vi "SDF Small Gasifier RT - IO_backup.vi"(0 "CIE Tags":T1) -> ()   [LabVIEW 2013]
uses:
  <userlib>/CIE/_TypeDefs/CIE Tags.ctl
  <userlib>/CIE/_TypeDefs/DBL CIE Tag.ctl
  <userlib>/CIE/_TypeDefs/BOOL CIE Tag.ctl
  <userlib>/CIE/_TypeDefs/I32 CIE Tag.ctl
  <userlib>/CIE/_TypeDefs/Enum CIE Tag.ctl
  <userlib>/CIE/_TypeDefs/STR CIE Tag.ctl
  <vilib>/NI/Current Value Table/DataTypes/String_Read.vi
  <vilib>/NI/Current Value Table/DataTypes/Double_Read.vi
  <vilib>/NI/Current Value Table/DataTypes/Double_Write.vi
  <vilib>/NI/Current Value Table/DataTypes/Boolean_Write.vi
  <vilib>/NI/Current Value Table/Type to Enum.vi
  <vilib>/NI/Current Value Table/DataTypes/String_Type To Enum.vi
  <vilib>/NI/Current Value Table/DataTypes/Double_Type To Enum.vi
  <vilib>/NI/Current Value Table/DataTypes/Boolean_Type To Enum.vi
  <vilib>/NI/Current Value Table/FGVs/CVT Globals.vi
  <vilib>/NI/Current Value Table/FGVs/Tag Memory.vi
  <vilib>/NI/Current Value Table/Memory Block.vi
  <vilib>/NI/Current Value Table/DataTypes/String_Memory Block.vi
  <vilib>/NI/Current Value Table/DataTypes/Double_Memory Block.vi
  <vilib>/NI/Current Value Table/DataTypes/Boolean_Memory Block.vi
  <vilib>/NI/Current Value Table/Current Value Table.lvlib
panel:
  out "Missed Scan":bool
  out "Scan Error":errorcluster
  out "Value":string
  out "Numeric":dbl
  in  "Stop":bool
  out "Index":i32
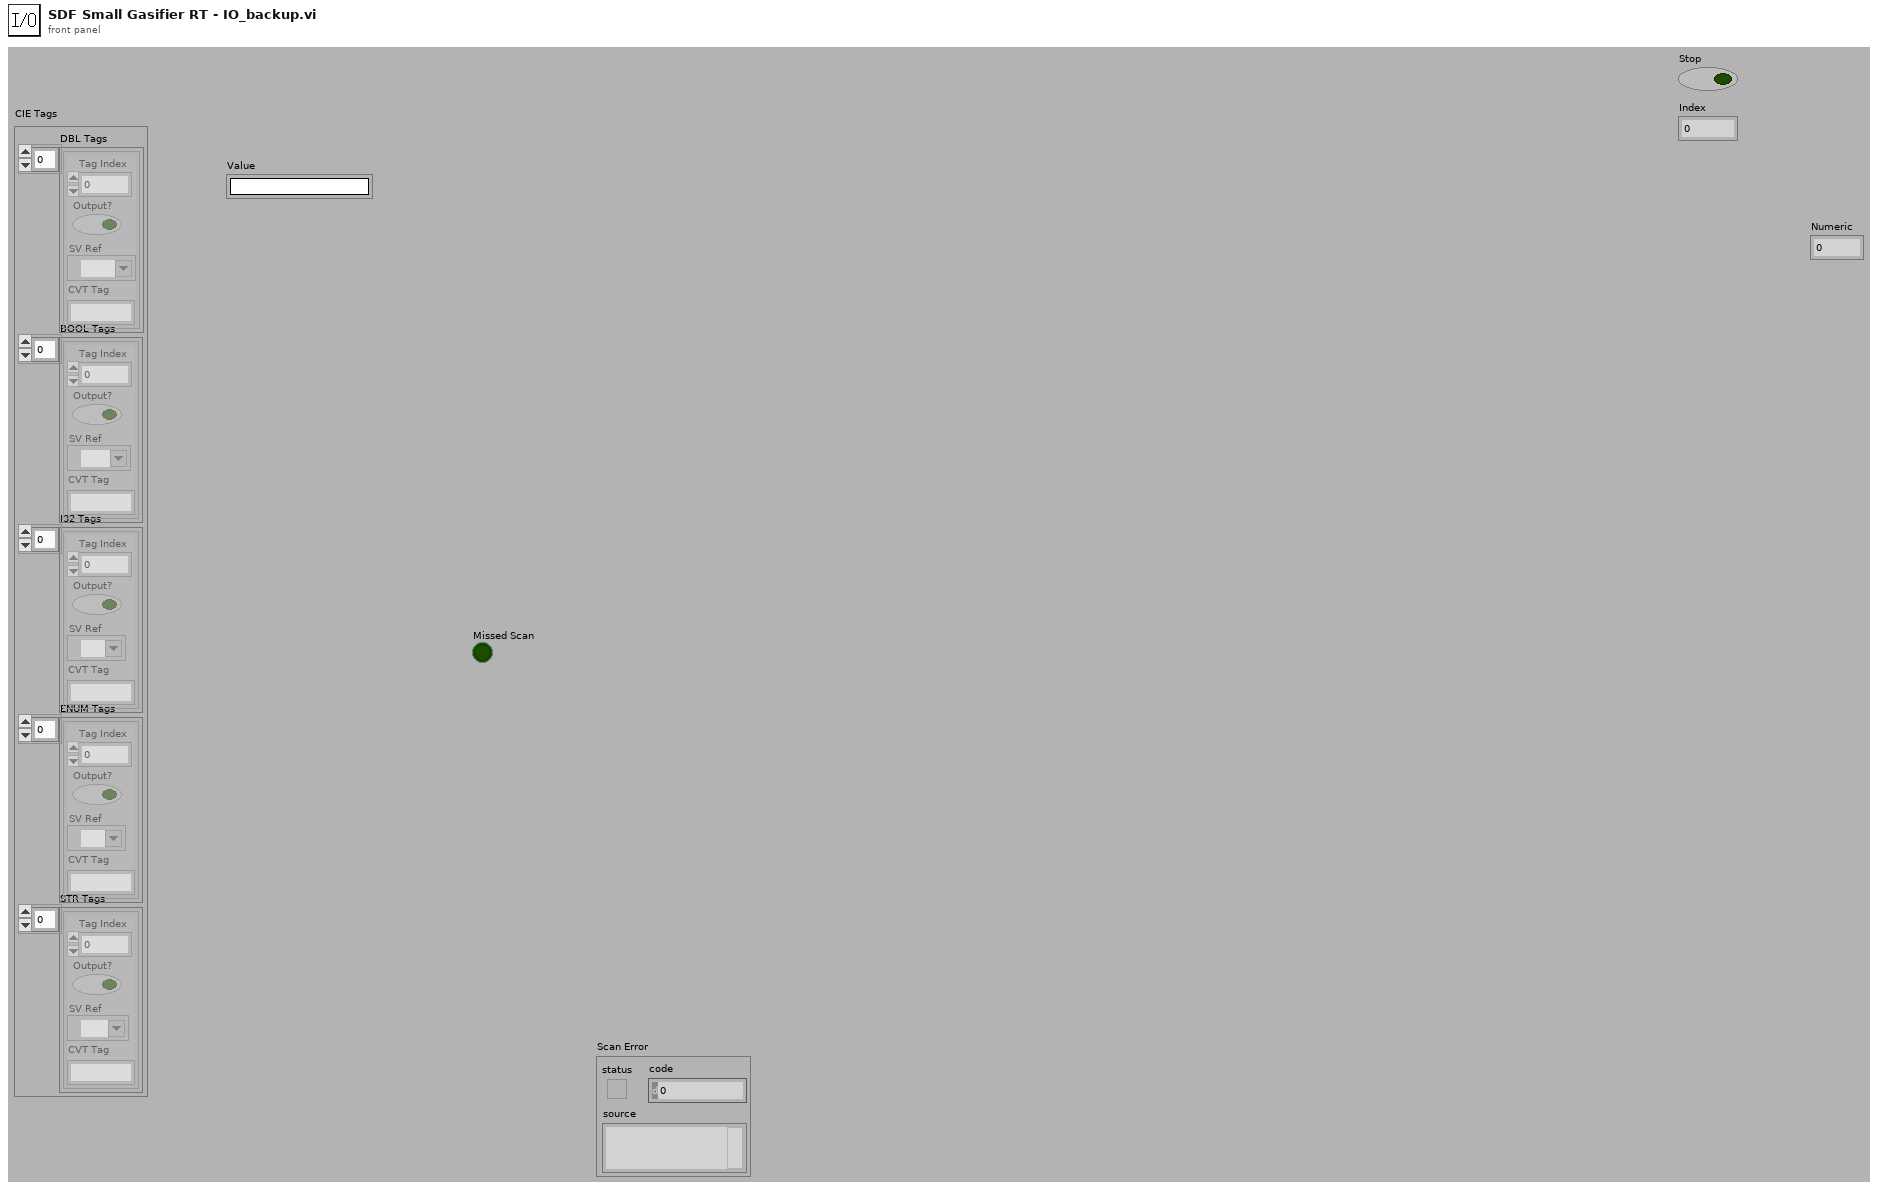
[diagram p1: front panel]
types:
  T1 = typedef "CIE Tags.ctl" = cluster{"DBL Tags":T2[], "BOOL Tags":T3[], "I32 Tags":T4[], "ENUM Tags":T5[], "STR Tags":T6[]}
  T2 = typedef "DBL CIE Tag.ctl" = cluster{"Tag Index":i32, "Output?":bool, "SV Ref":refnum<k21>, "CVT Tag":string}
  T3 = typedef "BOOL CIE Tag.ctl" = cluster{"Tag Index":i32, "Output?":bool, "SV Ref":refnum<k21>, "CVT Tag":string}
  T4 = typedef "I32 CIE Tag.ctl" = cluster{"Tag Index":i32, "Output?":bool, "SV Ref":refnum<k21>, "CVT Tag":string}
  T5 = typedef "Enum CIE Tag.ctl" = cluster{"Tag Index":i32, "Output?":bool, "SV Ref":refnum<k21>, "CVT Tag":string}
  T6 = typedef "STR CIE Tag.ctl" = cluster{"Tag Index":i32, "Output?":bool, "SV Ref":refnum<k21>, "CVT Tag":string}
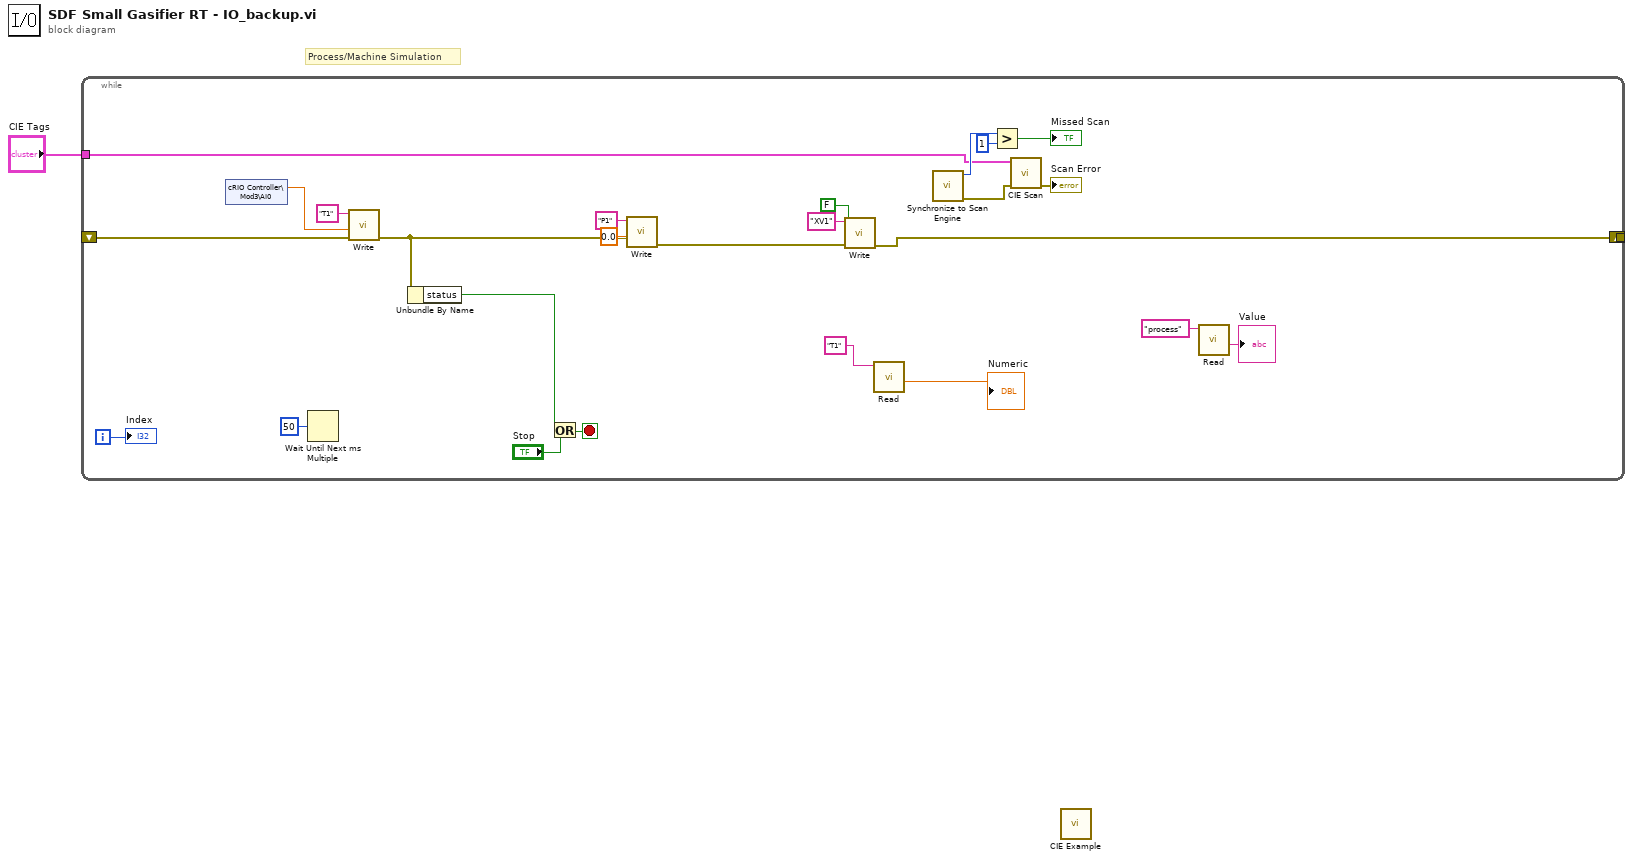
[diagram p0: block diagram]
diagram:
  # "Process/Machine Simulation"
  n1 = while {
    tunnel: [w10] -> _
    shift-right: [w10] -> _
    shift-left: _ -> [w21]
    tunnel: "CIE Tags" -> [w2]
    i -> [w25]
    stop <- w23 stop-if-true
    n2 = shared-variable "cRIO Controller\\Mod3\\AI0"() -> (w11:dbl)  [unwired: 1 in, 1 out]
    n3 = Wait Until Next ms Multiple(millisecond multiple=u32 50) -> ()  [unwired: 1 out]
    n4 = call-poly <vilib>:"Write.vi"("error in (no error)"=w21, "Value"=w11, "Tag Name"="T1") -> ("error out"=w15:errorcluster)  [unwired: 8 in]
    n5 = Unbundle By Name(w15) -> ("status"=w20:bool)
    n6 = Or(x=w20, y="Stop") -> (x .or. y?=w23:bool)
    n7 = call-poly <vilib>:"Write.vi"("error in (no error)"=w15, "Value"=0.0, "Tag Name"="P1") -> ("error out"=w14:errorcluster)  [unwired: 8 in]
    n8 = call-poly <vilib>:"Write.vi"("error in (no error)"=w14, "Value"=FALSE, "Tag Name"="XV1") -> ("error out"=w10:errorcluster)  [unwired: 8 in]
    n9 = call-poly <vilib>:"Read.vi"("Tag Name"="T1") -> ("Value"=→"Numeric":dbl)  [unwired: 9 in, 1 out]
    n10 = call <vilib>:"Synchronize to Scan Engine.vi"() -> ("error out"=w3:errorcluster, "scans since last call"=w5:u32)  [unwired: 10 in]
    n11 = Greater?(x=w5, y=u32 1) -> (0:→"Missed Scan":bool)
    n12 = call <userlib>:"CIE Scan.vi"("error in (no error)"=w3, "CIE Tags"=w2) -> ("error put"=→"Scan Error":errorcluster)  [unwired: 9 in]
    n13 = call-poly <vilib>:"Read.vi"("Tag Name"="process") -> ("Value"=→"Value":string)  [unwired: 9 in, 1 out]
    "Index" <- w25
  }
  n14 = call <userlib>:"CIE Example.vi"() -> ()  [unwired: 1 in]
